vi "PositionPlotInterval.vi"(8 "Reset":bool, 9 "Eta_d":dbl[](array[numeric]), 10 "Eta_e":dbl[](array[numeric]), 11 "Eta":dbl[](array[numeric])) -> ()   [LabVIEW 2014]
uses:
  Library/Helping Routines/Rad 2 PI-PI Vector.vi
panel:
  out "Waveform Chart 6":T1(graph)
  out "Waveform Chart 5":T1(graph)
  out "Waveform Chart 4":T1(graph)
  out "Waveform Chart 3":T1(graph)
  out "Waveform Chart 2":T1(graph)
  out "Waveform Chart":T1(graph)
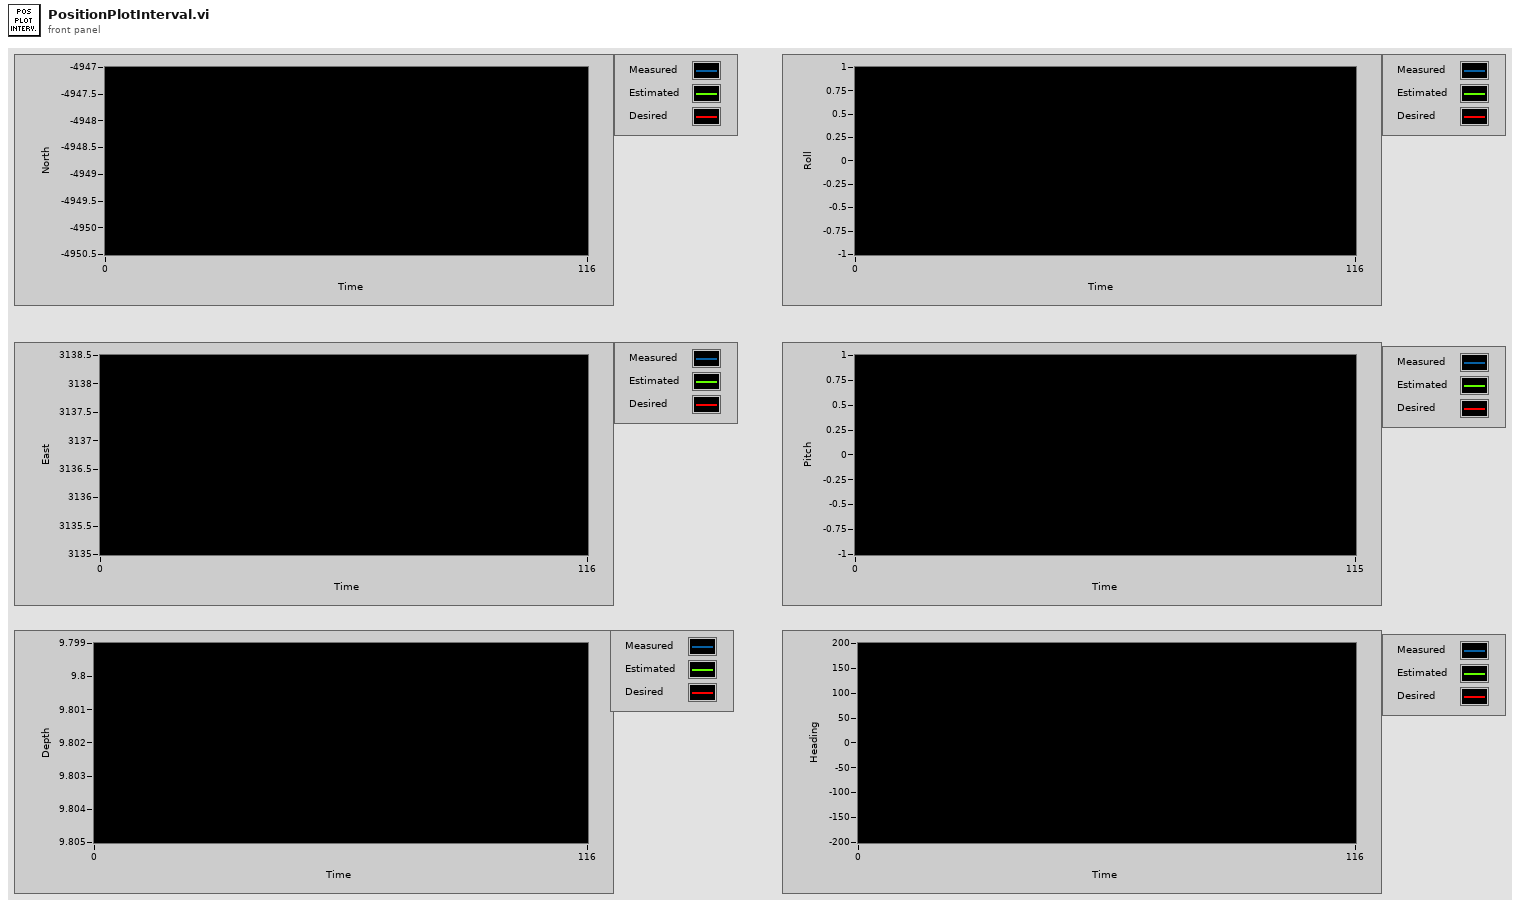
[diagram p1: front panel]
types:
  T1 = cluster{"Numeric":dbl, "Numeric":dbl, "Numeric":dbl}
  T2 = cluster{"Numeric":dbl, "Numeric":dbl, "Numeric":dbl}[]
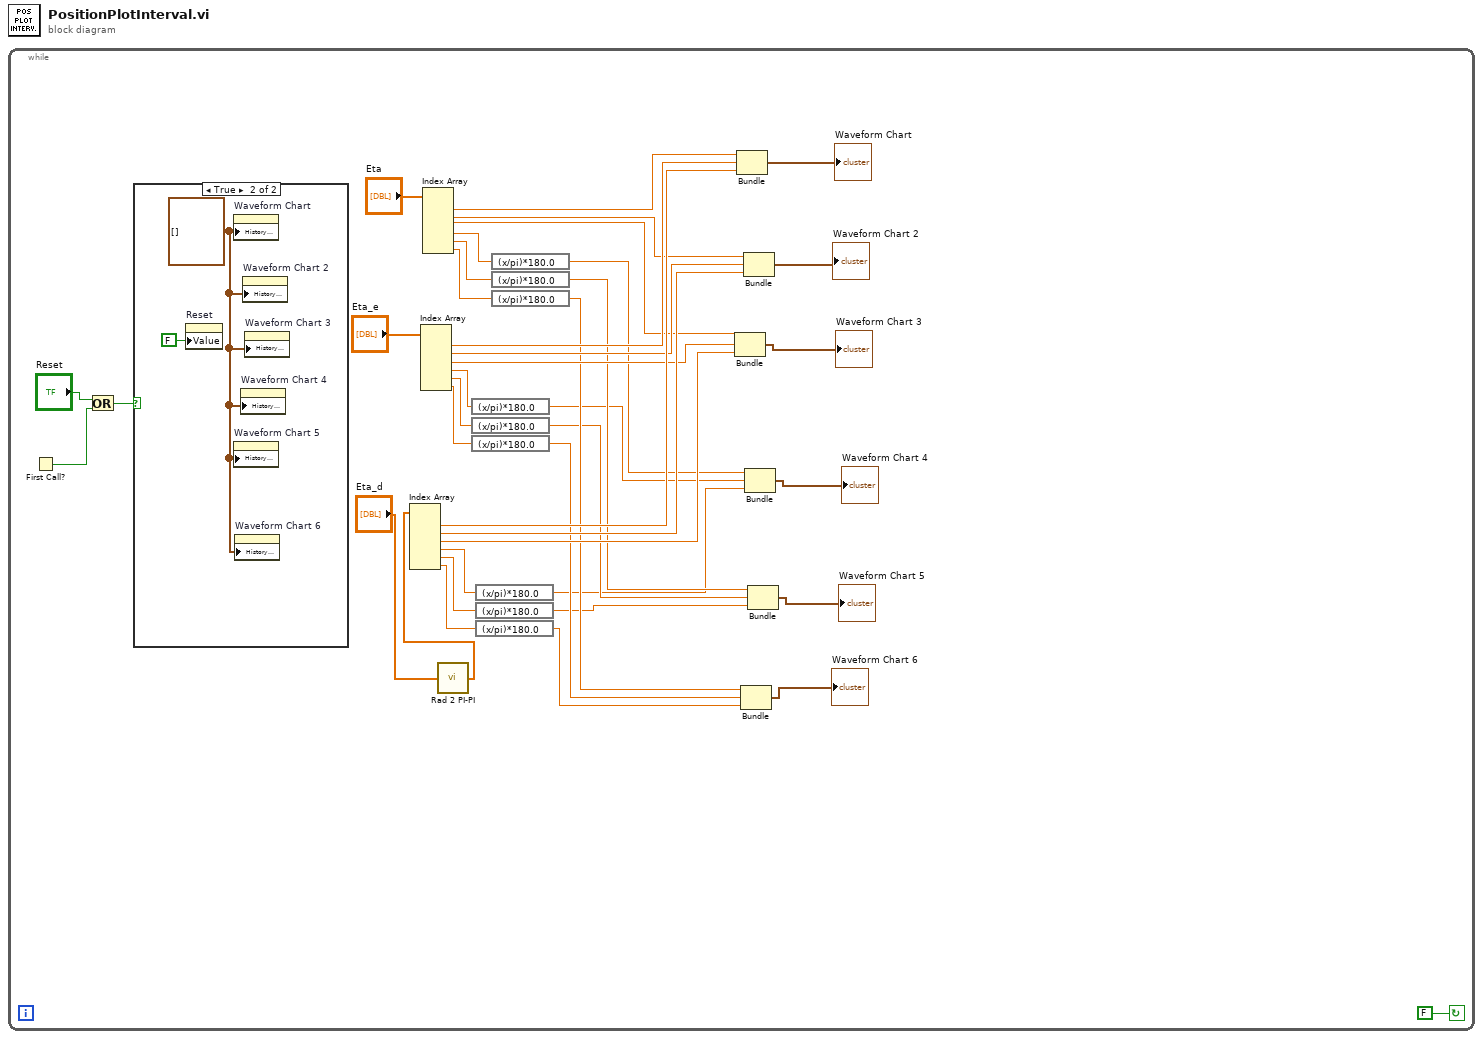
[diagram p0: block diagram]
diagram:
  n1 = while {
    stop <- FALSE continue-if-true
    n2 = First Call?() -> (First Call?: T/F=w21:bool)
    n3 = Or(x="Reset", y=w21) -> (x .or. y?=w23:bool)
    n4 = case shown="True" w23 {
      frame False {
      }
      frame True {
        w43 = T2 [] ("History Data")
        n5 = property on="Reset" class="Bool (strict)"("Value"=FALSE ("Reset")) -> ()  [unwired: 2 in, 2 out]
        n6 = property on="Waveform Chart" class="WFChart (strict)"("History Data"=w43) -> ()  [unwired: 2 in, 2 out]
        n7 = property on="Waveform Chart 5" class="WFChart (strict)"("History Data"=w43) -> ()  [unwired: 2 in, 2 out]
        n8 = property on="Waveform Chart 6" class="WFChart (strict)"("History Data"=w43) -> ()  [unwired: 2 in, 2 out]
        n9 = property on="Waveform Chart 4" class="WFChart (strict)"("History Data"=w43) -> ()  [unwired: 2 in, 2 out]
        n10 = property on="Waveform Chart 2" class="WFChart (strict)"("History Data"=w43) -> ()  [unwired: 2 in, 2 out]
        n11 = property on="Waveform Chart 3" class="WFChart (strict)"("History Data"=w43) -> ()  [unwired: 2 in, 2 out]
      }
    }
    n12 = Index Array(array="Eta_e") -> (element #1=w37:dbl, element #2=w33:dbl, element #3=w29:dbl, element #4=w10:dbl, element #5=w12:dbl, element #6=w14:dbl)  [unwired: 6 in]
    n13 = Index Array(array="Eta") -> (element #1=w38:dbl, element #2=w34:dbl, element #3=w30:dbl, element #4=w16:dbl, element #5=w18:dbl, element #6=w20:dbl)  [unwired: 6 in]
    n14 = call-poly "Rad 2 PI-PI.vi"("vector in"="Eta_d") -> ("vector out"=w1:dbl[])
    n15 = Index Array(array=w1) -> (element #1=w36:dbl, element #2=w32:dbl, element #3=w28:dbl, element #4=w8:dbl, element #5=w6:dbl, element #6=w4:dbl)  [unwired: 6 in]
    n16 = expression code="(x/pi)*180.0" ("radians to degrees")(w10) -> (w9:dbl)
    n17 = expression code="(x/pi)*180.0" ("radians to degrees")(w12) -> (w11:dbl)
    n18 = expression code="(x/pi)*180.0" ("radians to degrees")(w14) -> (w13:dbl)
    n19 = expression code="(x/pi)*180.0" ("radians to degrees")(w8) -> (w7:dbl)
    n20 = expression code="(x/pi)*180.0" ("radians to degrees")(w6) -> (w5:dbl)
    n21 = expression code="(x/pi)*180.0" ("radians to degrees")(w4) -> (w3:dbl)
    n22 = expression code="(x/pi)*180.0" ("radians to degrees")(w16) -> (w15:dbl)
    n23 = expression code="(x/pi)*180.0" ("radians to degrees")(w18) -> (w17:dbl)
    n24 = expression code="(x/pi)*180.0" ("radians to degrees")(w20) -> (w19:dbl)
    n25 = Bundle("Numeric"=w30, "Numeric"=w29, w28) -> (→"Waveform Chart 3":cluster{"Numeric":dbl, "Numeric":dbl, dbl})  [unwired: 1 in]
    n26 = Bundle("Numeric"=w38, "Numeric"=w37, w36) -> (→"Waveform Chart":cluster{"Numeric":dbl, "Numeric":dbl, dbl})  [unwired: 1 in]
    n27 = Bundle("Numeric"=w19, "Numeric"=w13, w3) -> (→"Waveform Chart 6":cluster{"Numeric":dbl, "Numeric":dbl, dbl})  [unwired: 1 in]
    n28 = Bundle("Numeric"=w34, "Numeric"=w33, w32) -> (→"Waveform Chart 2":cluster{"Numeric":dbl, "Numeric":dbl, dbl})  [unwired: 1 in]
    n29 = Bundle("Numeric"=w15, "Numeric"=w9, w7) -> (→"Waveform Chart 4":cluster{"Numeric":dbl, "Numeric":dbl, dbl})  [unwired: 1 in]
    n30 = Bundle("Numeric"=w17, "Numeric"=w11, w5) -> (→"Waveform Chart 5":cluster{"Numeric":dbl, "Numeric":dbl, dbl})  [unwired: 1 in]
  }
